vi "readBuffer.vi"(8 "error in (no error)":errorcluster, 11 "ElectrometerController in":refnum<class "ElectrometerController.lvclass">) -> (0 "error out":errorcluster, 3 "ElectrometerController out":refnum<class "ElectrometerController.lvclass">)   [LabVIEW 2016, in "ElectrometerController.lvclass"]
uses:
  ElectrometerController.lvclass
  ElectrometerController.lvclass/ElectrometerController.ctl
  ts_electrometeruserevents/ElectrometerProcessEvent/ElectrometerProcessEvent.lvclass/ElectrometerProcessEvent.ctl
  ts_electrometeruserevents/ElectrometerProcessEvent/ElectrometerProcessEvent.lvclass
  Electrometer/Electrometer.lvclass
  ElectrometerReading/ElectrometerReadingStatus.lvclass
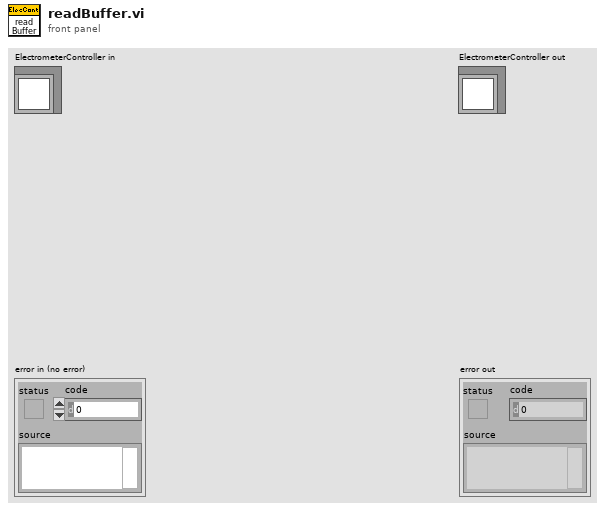
[diagram p1: front panel]
types:
  T1 = typedef "MiddlewareProcessEvents.ctl" = cluster{"disconnect":refnum<user-event>, "error":refnum<user-event>}
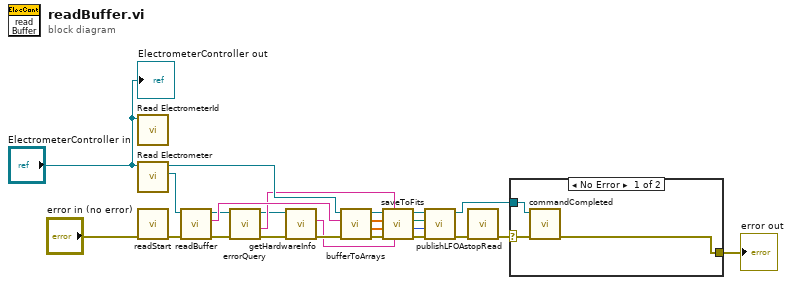
[diagram p0: block diagram]
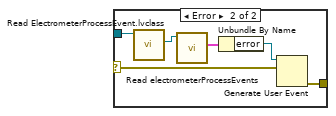
[diagram p2: hidden frame]
diagram:
  n1 = call-dynamic "Read ElectrometerId.vi"("ElectrometerController in"="ElectrometerController in") -> ()  [unwired: 8 in, 3 out]
  n2 = call-dynamic "Read Electrometer.vi"("ElectrometerController in"="ElectrometerController in") -> ("Electrometer.lvclass"=w25:refnum<class "Electrometer.lvclass">, "ElectrometerController out"=w21:refnum<class "ElectrometerController.lvclass">)  [unwired: 8 in, 1 out]
  n3 = call "readStart.vi"("error in (no error)"="error in (no error)") -> ("error out"=w23:errorcluster)  [unwired: 9 in, 1 out]
  n4 = call "readBuffer.vi"("error in (no error)"=w23, "Electrometer in"=w25) -> ("error out"=w10:errorcluster, "data"=w20:string, "Electrometer out"=w11:refnum<class "Electrometer.lvclass">)  [unwired: 7 in]
  n5 = call "errorQuery.vi"("error in (no error)"=w10, "Electrometer in"=w11) -> ("error out"=w8:errorcluster, "Error Message"=w9:string, "Electrometer out"=w6:refnum<class "Electrometer.lvclass">)  [unwired: 6 in, 1 out]
  n6 = call "getHardwareInfo.vi"("error in (no error)"=w8, "Electrometer in"=w6) -> ("error out"=w7:errorcluster, "electrometerInfo"=w5:string)  [unwired: 7 in, 1 out]
  n7 = call "bufferToArrays.vi"("error in (no error)"=w7, "BufferString"=w20, "ElectrometerController in"=w21) -> ("error out"=w18:errorcluster, "time"=w16:dbl[], "value"=w17:dbl[], "ElectrometerController out"=w19:refnum<class "ElectrometerController.lvclass">)  [unwired: 4 in, 1 out]
  n8 = call "saveToFits.vi"("hwInfo"=w5, "errorList"=w9, "error in (no error)"=w18, "time"=w16, "value"=w17, "ElectrometerController in"=w19) -> ("error out"=w14:errorcluster, "fileSize"=w12:i64, "Path"=w1:path, "ElectrometerController out"=w15:refnum<class "ElectrometerController.lvclass">)  [unwired: 2 in]
  n9 = call "publishLFOA.vi"("error in (no error)"=w14, "Byte_Size"=w12, "path"=w1, "ElectrometerController in"=w15) -> ("error out"=w13:errorcluster, "ElectrometerController out"=w3:refnum<class "ElectrometerController.lvclass">)  [unwired: 6 in]
  n10 = call "stopRead.vi"("error in (no error)"=w13) -> ("error out"=w2:errorcluster)  [unwired: 9 in, 1 out]
  n11 = case shown="No Error" w2 {
    selector: w2 -> [w28 w29]
    tunnel: [w26 w30] -> w4
    tunnel: w3 -> [w27 w34]
    frame No Error {
      n12 = call "commandCompleted.vi"("error in (no error)"=w28, "ElectrometerController in"=w27) -> ("error out"=w26:errorcluster)  [unwired: 8 in, 1 out]
    }
    frame Error {
      n13 = call "Read ElectrometerProcessEvent.lvclass.vi"("ElectrometerController in"=w34) -> ("ElectrometerProcessEvent.lvclass"=w33:refnum<class "ElectrometerProcessEvent.lvclass">)  [unwired: 8 in, 2 out]
      n14 = call "Read electrometerProcessEvents.vi"("MiddlewareProcessEvent in"=w33) -> ("MiddlewareProcessEvents"=w32:T1)  [unwired: 9 in, 1 out]
      n15 = Unbundle By Name(w32) -> ("error"=w31:refnum<user-event>)
      n16 = Generate User Event(user event=w31, event data cluster=w29) -> (error out=w30:errorcluster)  [unwired: 2 in, 1 out]
    }
  }
  "error out" <- w4
  "ElectrometerController out" <- "ElectrometerController in"
